vi "Read JSON Config.vi"(8 "error in (no error)":errorcluster, 10 "JSON Config":string, 11 "Subset_STR in":refnum<class "Insert_STR.lvclass">) -> (0 "error out":errorcluster, 3 "Subset_STR out":refnum<class "Insert_STR.lvclass">)   [LabVIEW 2021, in "Insert_STR.lvclass"]
uses:
  Insert_STR.lvclass
  Abs_Types/String/Abs_String.lvclass
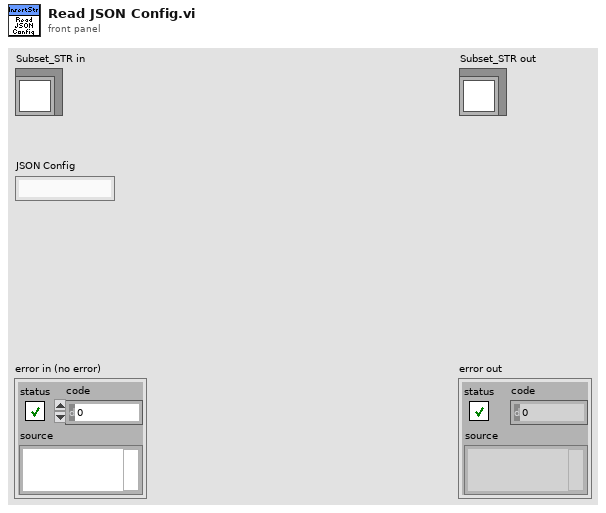
[diagram p1: front panel]
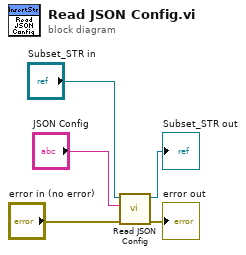
[diagram p0: block diagram]
diagram:
  n1 = call-parent "Read JSON Config.vi"("error in (no error)"="error in (no error)", "JSON Config"="JSON Config", "Abs_Type in"="Subset_STR in") -> ("error out"=→"error out":errorcluster, "Abs_Type out"=→"Subset_STR out":refnum<class "Insert_STR.lvclass">)  [unwired: 7 in]
